vi "file to matrix.vi"(9 "number format (%.3f)":string="%le", 10 "File Path":path=path "E:/data4/MF.txt", 11 "number of rows (all:-1)":i32=-1) -> (3 "all rows":dbl[][](array[numeric]) format="%0.3f")   [LabVIEW 2012, in "LightPipes.lvlib"]
uses:
  LightPipes.lvlib
  <vilib>/Utility/file.llb/Read From Spreadsheet File (DBL).vi
panel:
  out "Image":T1(plugin-control)
  out "Intensity Graph":dbl[][](graph)
  in  "delimiter (\\t)":string="  "
  in  "max characters/row  (no limit:0)":i32
  out "EOF?":bool
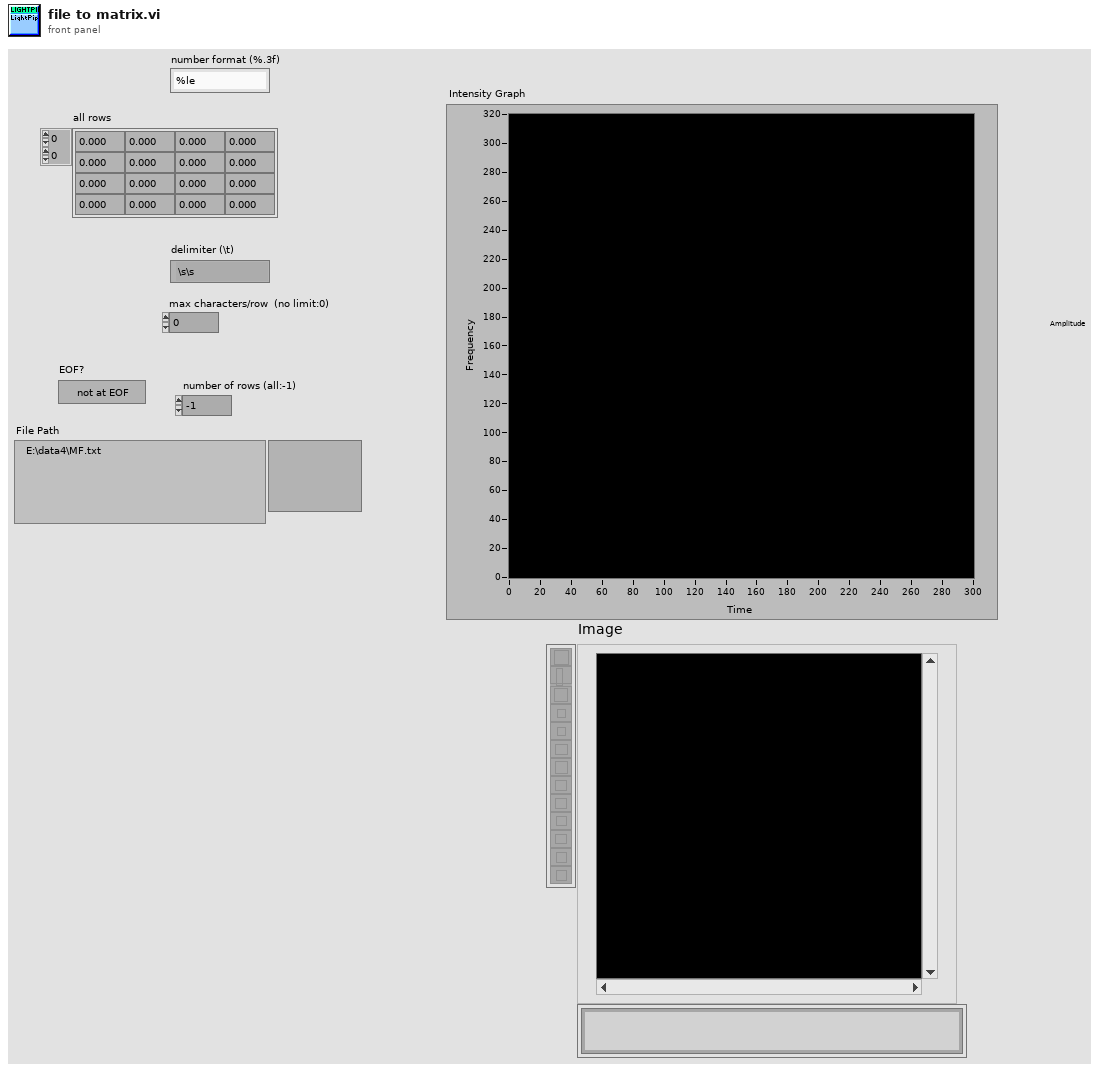
[diagram p1: front panel]
types:
  T1 = typedef "IMAQ Image.ctl" = refnum<image>
  T2 = typedef "Image Type" = u32
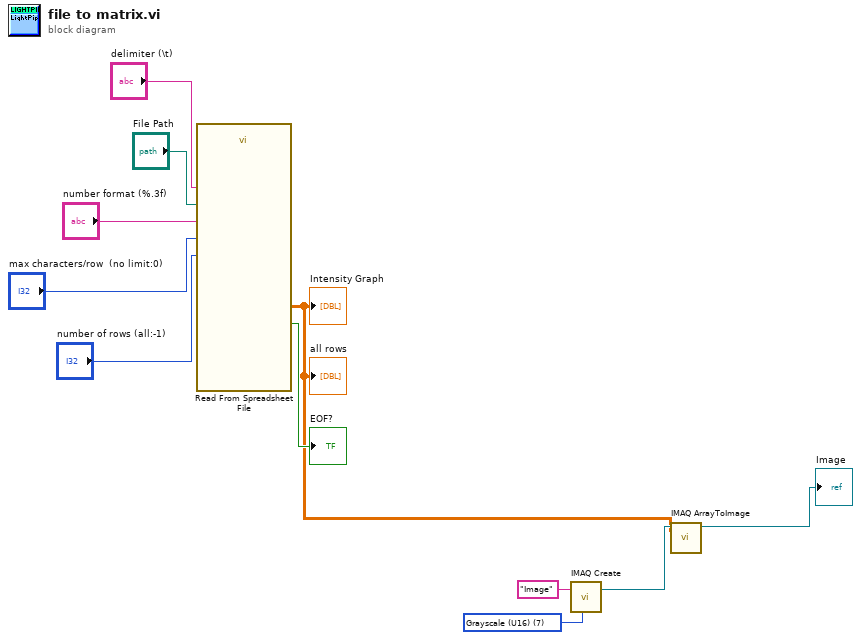
[diagram p0: block diagram]
diagram:
  w2 = T2 7 items=["Grayscale (U8)", "Grayscale (I16)", "Grayscale (SGL)", "Complex (CSG)", "RGB (U32)", "HSL (U32)", "RGB (U64)", "Grayscale (U16)"] ("Image Type")
  n1 = call-poly <vilib>:"Read From Spreadsheet File.vi"("delimiter (\\t)"="delimiter (\\t)", "format (%.3f)"="number format (%.3f)", "max characters/row  (no limit:0)"="max characters/row  (no limit:0)", "number of rows (all:-1)"="number of rows (all:-1)", "file path (dialog if empty)"="File Path") -> ("EOF?"=→"EOF?":bool, "all rows"=w1:dbl[][])  [unwired: 2 in, 3 out]
  "all rows" <- w1
  "Intensity Graph" <- w1
  n2 = call "IMAQ Create"("Image Name"="Image", "Image Type"=w2) -> ("New Image"=w4:T1)  [unwired: 3 in, 1 out]
  n3 = call "IMAQ ArrayToImage"("Image Pixels (U16)"=w1, "Image"=w4) -> ("Image Out"=→"Image":T1)  [unwired: 8 in, 1 out]
